vi "Sequence.CreateConditions.vi"(8 "error in (no error)":errorcluster, 9 "Condition":T1, 10 "Iteration":string, 11 "Task":refnum<k24>) -> (0 "error out":errorcluster, 3 "Tasks":refnum<k24>[](array[refnum]))   [LabVIEW 2013, in "Simple Sequence Editor.lvlib"]
uses:
  Simple Sequence Editor.lvlib
  NationalInstruments.VeriStand.RealTimeSequenceDefinitionApi
  Types/Compiled.StepCondition.ctl
  Types/OperationTypes.ctl
  Constants.vi
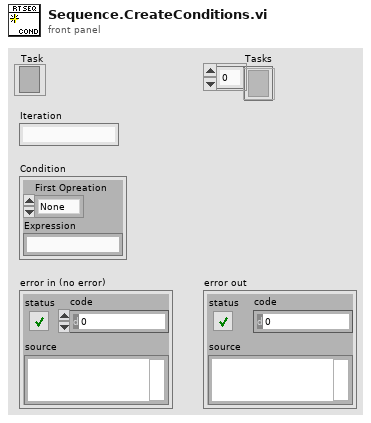
[diagram p1: front panel]
types:
  T1 = typedef "Simple Sequence Editor.lvlib/Compiled.StepCondition.ctl" = cluster{"First Opreation":T2, "Expression":string}
  T2 = typedef "Simple Sequence Editor.lvlib/OperationTypes.ctl" = enum8{"None", "&&", "||"}
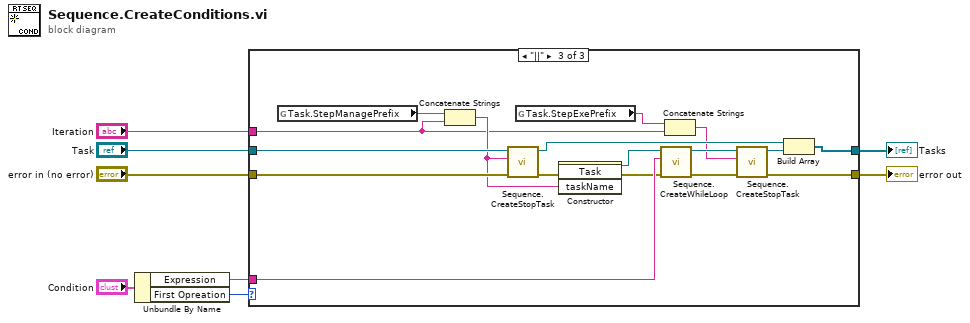
[diagram p0: block diagram]
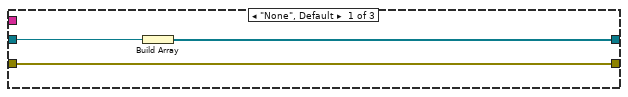
[diagram p2: hidden frame]
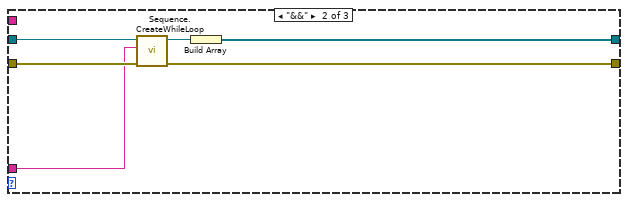
[diagram p3: hidden frame]
diagram:
  n1 = Unbundle By Name("Condition") -> ("Expression"=w5:string, "First Opreation"=w4:T2)
  n2 = case shown="\"||\"" w4 {
    tunnel: [w9 w12 w22] -> w7
    tunnel: "error in (no error)" -> [w9 w17 w26]
    tunnel: "Task" -> [w11 w16 w28]
    tunnel: "Iteration" -> [_ _ w20]
    tunnel: w5 -> [_ w15 w34]
    tunnel: [w10 w13 w23] -> w6
    frame "None", Default {
      n3 = Build Array(w11) -> (w10:refnum<k24>[])
    }
    frame "&&" {
      n4 = call "Sequence.CreateWhileLoop.vi"("error in (no error)"=w17, "Expression"=w15, "Task Ref"=w16) -> ("error out"=w12:errorcluster, "Task Ref out"=w14:refnum<k24>)  [unwired: 7 in]
      n5 = Build Array(w14) -> (w13:refnum<k24>[])
    }
    frame "||" {
      n6 = global read "Constants.vi" "Task.StepManagePrefix"() -> (w18:string)
      n7 = Concatenate Strings(w18, w20) -> (w24:string)
      n8 = call "Sequence.CreateStopTask.vi"("error in (no error)"=w26, "Task Name"=w24, "Task Ref"=w28) -> ("error out"=w25:errorcluster, ".NET Refnum out"=w27:refnum<k24>)  [unwired: 7 in]
      n9 = global read "Constants.vi" "Task.StepExePrefix"() -> (w21:string)
      n10 = constructor class="Task"(error in=w25, "taskName"=w24) -> (reference out=w33:refnum<k24>, error out=w32:errorcluster)  [unwired: 2 in, 2 out]
      n11 = call "Sequence.CreateWhileLoop.vi"("error in (no error)"=w32, "Expression"=w34, "Task Ref"=w33) -> ("error out"=w29:errorcluster, "Task Ref out"=w31:refnum<k24>)  [unwired: 7 in]
      n12 = Concatenate Strings(w21, w20) -> (w19:string)
      n13 = call "Sequence.CreateStopTask.vi"("error in (no error)"=w29, "Task Name"=w19, "Task Ref"=w31) -> ("error out"=w22:errorcluster, ".NET Refnum out"=w30:refnum<k24>)  [unwired: 7 in]
      n14 = Build Array(w27, w30) -> (w23:refnum<k24>[])
    }
  }
  "error out" <- w7
  "Tasks" <- w6
